vi "get terminal info.vi"(8 "error in (no error)":errorcluster, 10 "Get Object Terminals Argument":T2, 11 "Data Cluster in":T1) -> (0 "error out":errorcluster, 2 "String":string, 3 "Data Cluster out":T1)   [LabVIEW 2025, in "Scripting Server.lvlib"]
uses:
  Scripting Server.lvlib
  Module Data--cluster.ctl
  Get Object Terminals Argument--cluster.ctl
  Get Object Terminals (Reply Payload)--cluster.ctl
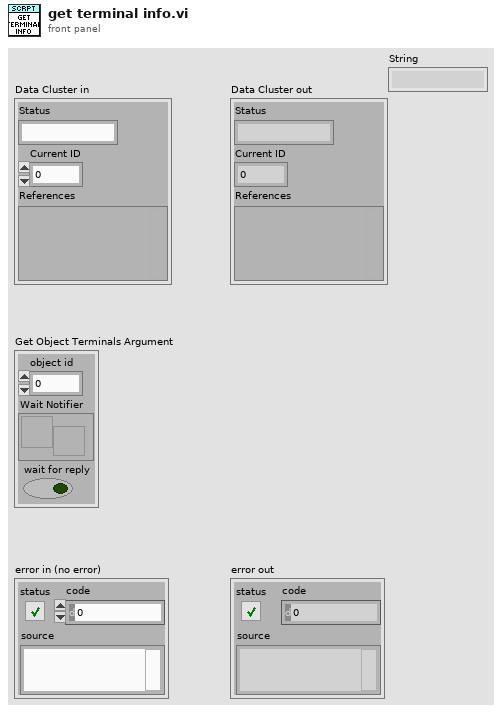
[diagram p1: front panel]
types:
  T1 = typedef "Scripting Server.lvlib/Module Data--cluster.ctl" = cluster{"Status":string, "Current ID":i32, "References":variant}
  T2 = typedef "Scripting Server.lvlib/Get Object Terminals Argument--cluster.ctl" = cluster{"object id":i32, "Wait Notifier":refnum<notifier>, "wait for reply":bool}
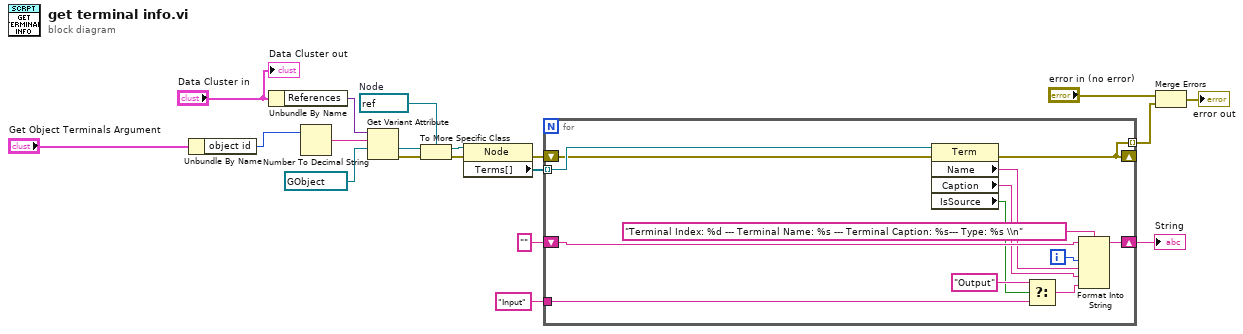
[diagram p0: block diagram]
diagram:
  w7 = refnum<vi> refnum  # Node
  n1 = Unbundle By Name("Get Object Terminals Argument") -> ("object id"=w14:i32)
  n2 = Unbundle By Name("Data Cluster in") -> ("References"=w15:variant)
  n3 = Number To Decimal String(number=w14) -> (decimal integer string=w13:string)  [unwired: 1 in]
  n4 = Get Variant Attribute(Variant=w15, name=w13, default value (empty Variant)=refnum<vi> refnum ("reference")) -> (value=w9:refnum<vi>, error out=w11:errorcluster)  [unwired: 1 in, 2 out]
  n5 = To More Specific Class(target class=w7, reference=w9, error in=w11) -> (specific class reference=w8:refnum<vi>, error out=w10:errorcluster)
  n6 = property class="Node"(reference=w8, error in=w10) -> (error out=w4:errorcluster, "Terms[]"=w5:refnum<vi>[])  [unwired: 1 out]
  n7 = for {
    shift-right: [w31] -> w3
    shift-left: "" -> [w32]
    tunnel: w5 -> [w28] mode=indexing
    shift-right: [w24] -> _
    shift-left: w4 -> [w27]
    tunnel: [w24] -> w2 mode=indexing
    tunnel: "Input" ("input 4") -> [w21]
    i -> [w29]
    n8 = property class="Term"(reference=w28, error in=w27) -> (error out=w24:errorcluster, "Name"=w26:string, "Caption"=w25:string, "IsSource"=w20:bool)  [unwired: 1 out]
    n9 = Select(t="Output" ("input 4"), s=w20, f=w21) -> (s? t:f=w22:string)
    n10 = Format Into String(format string="Terminal Index: %d --- Terminal Name: %s --- Terminal Caption: %s--- Type: %s \\n", initial string=w32, w29, w26, w25, w22) -> (resulting string=w31:string)  [unwired: 1 in, 1 out]
  }
  "String" <- w3
  n11 = Merge Errors("error in (no error)", w2) -> (→"error out":errorcluster)
  "Data Cluster out" <- "Data Cluster in"
